vi "Set Size.vi"(8 "error in (no error)":errorcluster, 9 "Widht":u32, 10 "Height":u32, 11 "TabControlRef in":refnum<vi>) -> (0 "error out":errorcluster, 3 "TabControlRef out":refnum<vi>)   [LabVIEW 2020, in "MDI ViewManager.lvlib"]
uses:
  MDI ViewManager.lvlib
  <vilib>/Utility/miscctls.llb/LVBoundsTypeDef.ctl
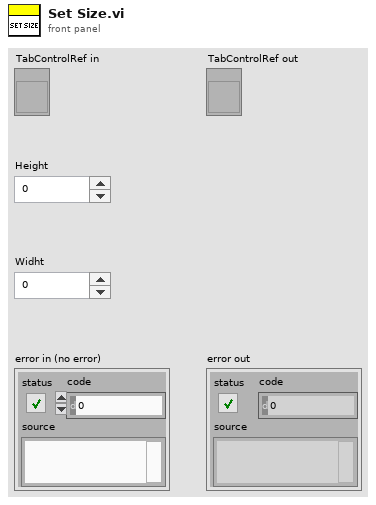
[diagram p1: front panel]
types:
  T1 = typedef "LVBoundsTypeDef.ctl" = cluster{"Width":u32, "Height":u32}
  T2 = typedef "LVPositionTypeDef.ctl" = cluster{"Left":i32, "Top":i32}
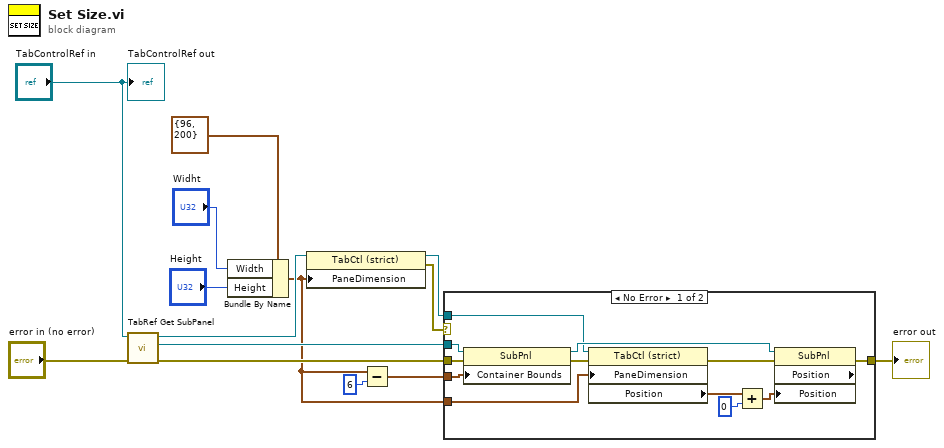
[diagram p0: block diagram]
diagram:
  n1 = call "TabRef Get SubPanel.vi"("error in (no error)"="error in (no error)", "TabControl in"="TabControlRef in") -> ("error out"=w10:errorcluster, "Sub Panel"=w14:refnum<vi>, "TabControl out"=w7:refnum<vi>)  [unwired: 7 in]
  n2 = Bundle By Name(cluster=T1 {"Width"=96, "Height"=200} ("TabDimension"), "Width"="Widht", "Height"="Height") -> (w6:T1)
  n3 = property class="TabCtl (strict)"(reference=w7, "PaneDimension"=w6) -> (reference out=w2:refnum<vi>, error out=w5:errorcluster)  [unwired: 1 in]
  n4 = Subtract(x=w6, y=6) -> (x-y=w8:T1)
  n5 = case shown="No Error" w5 {
    selector: w5 -> [_ w27]
    tunnel: w14 -> [w26 _]
    tunnel: w10 -> [w24 _]
    tunnel: w8 -> [w19 _]
    tunnel: w2 -> [w18 _]
    tunnel: w6 -> [w17 _]
    tunnel: [w16 w27] -> w4
    frame No Error {
      n6 = property class="SubPnl"(reference=w26, error in=w24, "Container Bounds"=w19) -> (reference out=w23:refnum<vi>, error out=w25:errorcluster)
      n7 = property class="TabCtl (strict)"(reference=w18, error in=w25, "PaneDimension"=w17) -> (error out=w22:errorcluster, "Position"=w21:T2)  [unwired: 1 out]
      n8 = Add(x=w21, y=0) -> (x+y=w20:T2)
      n9 = property class="SubPnl" props=["Position", "Position"](reference=w23, error in=w22, "Position"=w20) -> (error out=w16:errorcluster)  [unwired: 2 out]
    }
    frame Error {
    }
  }
  "error out" <- w4
  "TabControlRef out" <- "TabControlRef in"
